vi "Bulk Mode Read Data.vi"(7 "SlaveID":u8=1, 8 "error in (no error)":errorcluster, 9 "# samples to read":u16, 11 ".NET Refnum in":refnum<k24>) -> (0 "error out":errorcluster, 1 "# samples in buffer":u16, 2 "Vib":u16[](array[numeric]), 3 "reference out":refnum<k24>)   [LabVIEW 2017]
uses:
  C:/Users/chrisjan/Desktop/NowWorking/ITRI/DLL/Modbus.dll
  DLL/Modbus.dll
panel:
  out "-1 = Normal Mode":i16
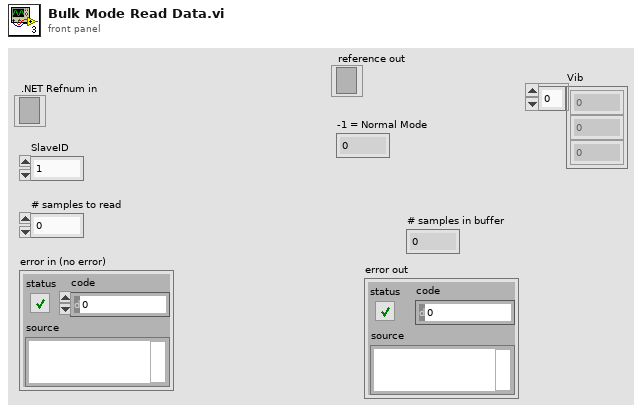
[diagram p1: front panel]
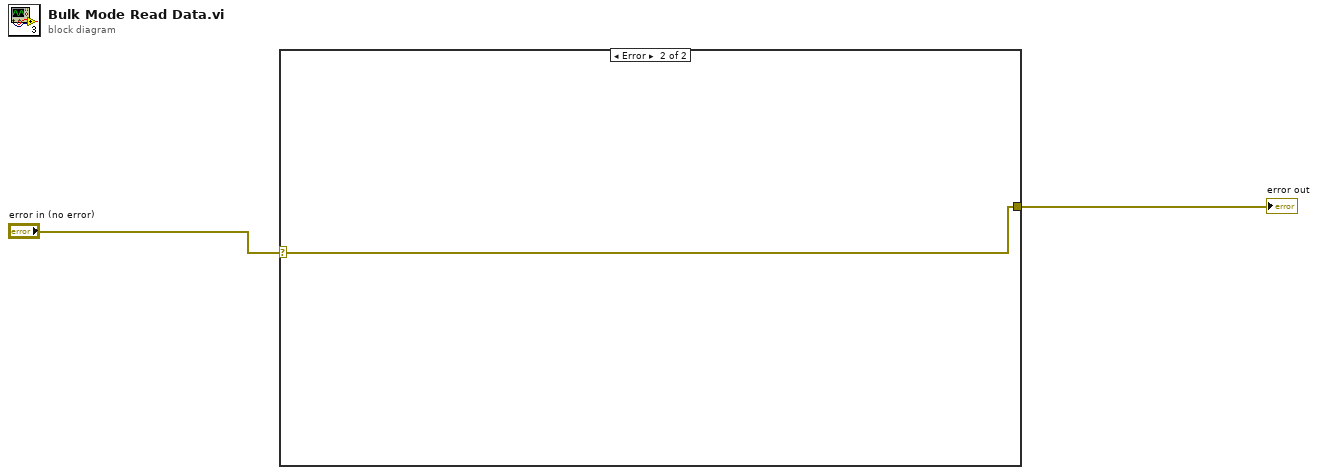
[diagram p0: block diagram]
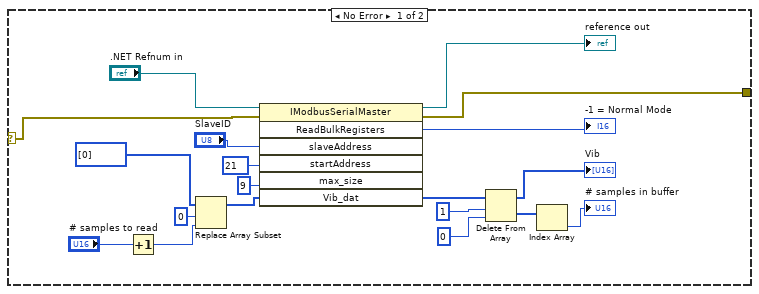
[diagram p2: hidden frame]
diagram:
  n1 = case shown="Error" "error in (no error)" {
    selector: "error in (no error)" -> [w3 w22]
    tunnel: [w15 w22] -> w2
    frame No Error {
      n2 = Increment(x="# samples to read") -> (x+1=w12:u16)
      n3 = Replace Array Subset(array=u16[] [0], new element=w12, index=0) -> (w9:u16[])
      n4 = invoke class="IModbusSerialMaster" method="ReadBulkRegisters"(reference=".NET Refnum in", error in=w3, "slaveAddress"="SlaveID", "startAddress"=u16 21, "max_size"=i16 9, "Vib_dat"=w9) -> (reference out=→"reference out":refnum<k24>, error out=w15:errorcluster, "ReadBulkRegisters"=→"-1 = Normal Mode":i16, "Vib_dat"=w8:u16[])  [unwired: 1 in, 3 out]
      n5 = Delete From Array(array=w8, length=1, index=0) -> (deleted portion=w7:u16[], array with subset deleted=→"Vib":u16[])
      n6 = Index Array(array=w7) -> (element=→"# samples in buffer":u16)  [unwired: 1 in]
    }
    frame Error {
    }
  }
  "error out" <- w2
